vi "LoadCfgXMLFile.vi"(7 "ChassisType":T1, 8 "error in":errorcluster, 11 "XML File Path":path) -> (0 "error out":errorcluster, 3 "Chassis Cfg":refnum<class "ChassisCfg.lvclass">)   [LabVIEW 2012, in "Configuration Grandmaster.lvlib" / "ChassisCfg.lvclass"]
uses:
  ChassisCfg.lvclass
  Common/Controls/Chassis Type.ctl
  Common/Controls/LS Lock Sizes.ctl
  Custom Ctrls/Master CfgXML/ge_XMLHdr_TimingGrp.ctl
  Custom Ctrls/Master CfgXML/ge_XMLHdr_ChanGroups.ctl
  Custom Ctrls/Master Cfg/ge_GrpHdr.ctl
  Custom Ctrls/ge_MeasType.ctl
  ChassisCfg.lvclass/ChassisCfg.ctl
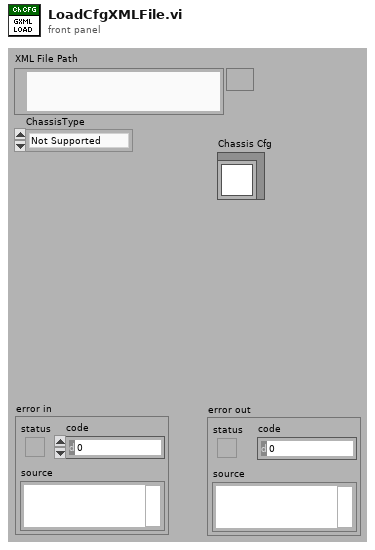
[diagram p1: front panel]
types:
  T1 = typedef "Chassis Type.ctl" = enum16{"Not Supported", "C Series 1-Slot", "C Series 4-Slot", "C Series 8-Slot", "PXI 8-Slot", "PXIe 18-Slot"}
  T2 = typedef "ge_XMLHdr_TimingGrp.ctl" = cluster{"Rate":dbl, "ReadBlk":i32, "Modbus URL":string, "ChanGroups":T3}
  T3 = typedef "ge_XMLHdr_ChanGroups.ctl" = T4[]
  T4 = typedef "ge_GrpHdr.ctl" = cluster{"GroupName":string, "MeasType":T5}
  T5 = typedef "ge_MeasType.ctl" = enum16{"Voltage", "Frequency", "Tachometer", "Dynamic", "Thermocouple", "RTD", "Strain", "Current", "Resistance"}
  T6 = typedef "LS Lock Sizes.ctl" = enum16{"No", "250ms", "500ms", "1s"}
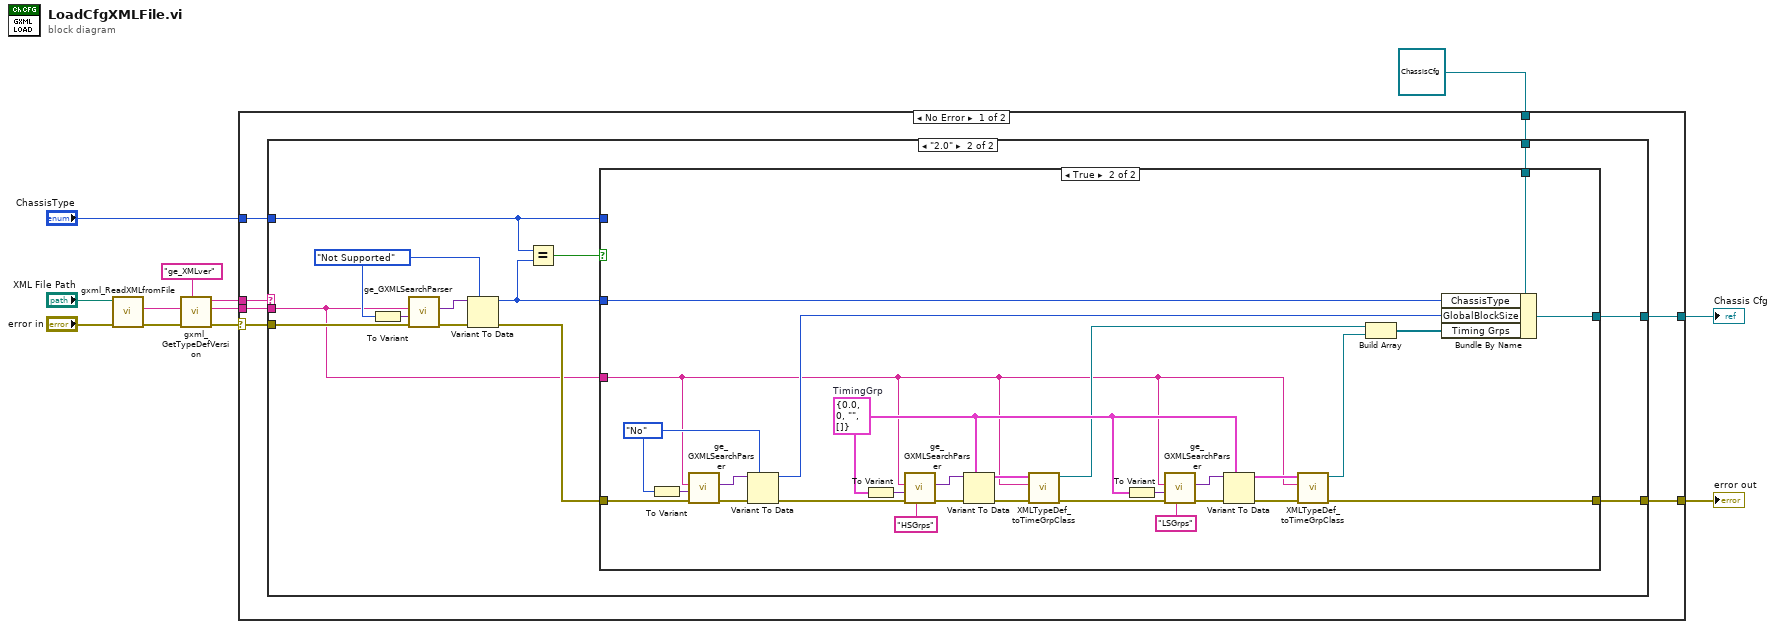
[diagram p0: block diagram]
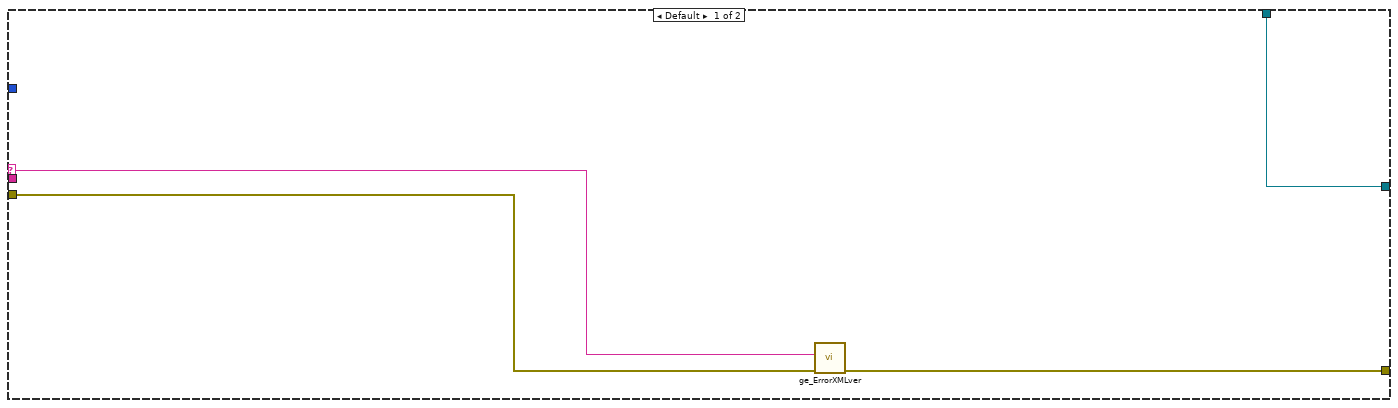
[diagram p2: hidden frame]
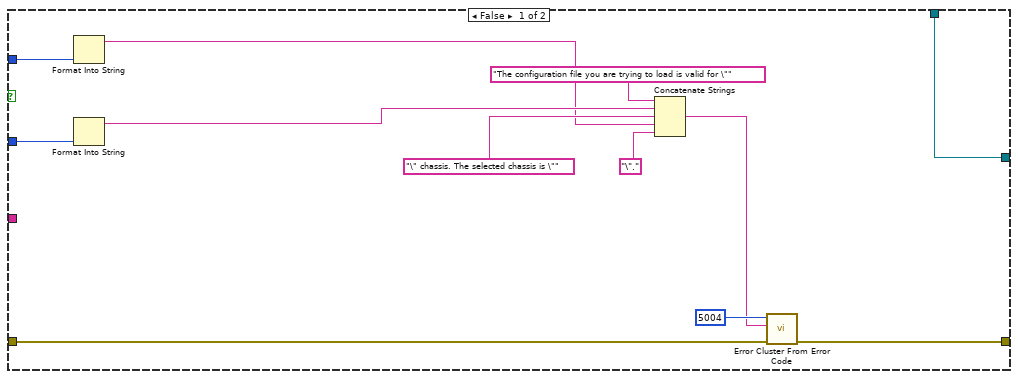
[diagram p3: hidden frame]
diagram:
  n1 = call <userlib>:"gxml_ReadXMLfromFile.vi"("error in"="error in", "XML File Path"="XML File Path") -> ("error out"=w8:errorcluster, "XML String Out"=w9:string)  [unwired: 7 in, 1 out]
  n2 = call <userlib>:"gxml_GetTypeDefVersion.vi"("Version Tag Name"="ge_XMLver", "error in"=w8, "XML String In"=w9) -> ("error out"=w5:errorcluster, "XML String Out"=w6:string, "Version String"=w4:string)  [unwired: 6 in]
  n3 = case shown="No Error" w5 {
    selector: w5 -> [w17 w79]
    tunnel: [w19 w78] -> w1
    tunnel: [w18 w79] -> w12
    tunnel: w6 -> [w14 _]
    tunnel: refnum<class "ChassisCfg.lvclass"> refnum ("Chassis Config") -> [w16 w78]
    tunnel: w4 -> [w15 _]
    tunnel: "ChassisType" -> [w13 _]
    frame No Error {
      n4 = case shown="\"2.0\"" w15 {
        selector: w15 -> [w20 _]
        tunnel: [w23 w36] -> w19
        tunnel: [w22 w35] -> w18
        tunnel: w17 -> [w21 w31]
        tunnel: w16 -> [w23 w34]
        tunnel: w14 -> [_ w27]
        tunnel: w13 -> [_ w25]
        frame Default {
          n5 = call "ge_ErrorXMLver.vi"("error in"=w21, "File Version Number"=w20) -> ("error out"=w22:errorcluster)  [unwired: 9 in]
        }
        frame "2.0" {
          w28 = Chassis_Type."Not Supported" ("ChassisType")
          n6 = To Variant(anything=w28) -> (Variant=w29:variant)
          n7 = call "ge_GXMLSearchParser.vi"("error in"=w31, "TypeDesc"=w29, "XML String In"=w27) -> ("error out"=w33:errorcluster, "Parsed Data"=w30:variant)  [unwired: 7 in]
          n8 = Variant To Data(error in=w33, type=w28, Variant=w30) -> (data=w24:T1, error out=w32:errorcluster)
          n9 = Equal?(x=w25, y=w24) -> (x = y?=w26:bool)
          n10 = case shown="True" w26 {
            tunnel: [w48 w77] -> w36
            tunnel: [w47 w50] -> w35
            tunnel: w34 -> [w48 w76]
            tunnel: w32 -> [w46 w75]
            tunnel: w24 -> [w43 w74]
            tunnel: w27 -> [_ w49]
            tunnel: w25 -> [w44 _]
            frame False {
              n11 = Format Into String(w44) -> (resulting string=w39:string)  [unwired: 3 in, 1 out]
              n12 = Format Into String(w43) -> (resulting string=w41:string)  [unwired: 3 in, 1 out]
              n13 = Concatenate Strings("The configuration file you are trying to load is valid for \"", w41, "\" chassis. The selected chassis is \"", w39, "\".") -> (w37:string)
              n14 = call <vilib>:"Error Cluster From Error Code.vi"("error in (no error)"=w46, "error message (\"\")"=w37, "error code (0)"=5004) -> ("error out"=w47:errorcluster)  [unwired: 6 in]
            }
            frame True {
              w59 = T2 {"Rate"=0.0, "ReadBlk"=0, "Modbus URL"="", "ChanGroups"=[]}  # TimingGrp
              w62 = LS_Lock_Sizes."No" ("GlobalBlockSize")
              n15 = To Variant(anything=w62) -> (Variant=w65:variant)
              n16 = call "ge_GXMLSearchParser.vi"("error in"=w75, "TypeDesc"=w65, "XML String In"=w49) -> ("error out"=w71:errorcluster, "Parsed Data"=w70:variant)  [unwired: 7 in]
              n17 = Variant To Data(error in=w71, type=w62, Variant=w70) -> (data=w61:T6, error out=w60:errorcluster)
              n18 = To Variant(anything=w59) -> (Variant=w63:variant)
              n19 = call "ge_GXMLSearchParser.vi"("String ID"="HSGrps", "error in"=w60, "TypeDesc"=w63, "XML String In"=w49) -> ("error out"=w69:errorcluster, "Parsed Data"=w68:variant)  [unwired: 6 in]
              n20 = Variant To Data(error in=w69, type=w59, Variant=w68) -> (data=w55:T2, error out=w56:errorcluster)
              n21 = call "XMLTypeDef_toTimeGrpClass.vi"("error in (no error)"=w56, "XML String"=w49, "TimingGrp"=w55) -> ("error out"=w54:errorcluster, "TimingGrp out"=w58:refnum<class "TimingGrp.lvclass">)  [unwired: 7 in]
              n22 = To Variant(anything=w59) -> (Variant=w64:variant)
              n23 = call "ge_GXMLSearchParser.vi"("String ID"="LSGrps", "error in"=w54, "TypeDesc"=w64, "XML String In"=w49) -> ("error out"=w66:errorcluster, "Parsed Data"=w67:variant)  [unwired: 6 in]
              n24 = Variant To Data(error in=w66, type=w59, Variant=w67) -> (data=w52:T2, error out=w53:errorcluster)
              n25 = call "XMLTypeDef_toTimeGrpClass.vi"("error in (no error)"=w53, "XML String"=w49, "TimingGrp"=w52) -> ("error out"=w50:errorcluster, "TimingGrp out"=w51:refnum<class "TimingGrp.lvclass">)  [unwired: 7 in]
              n26 = Build Array(w58, w51) -> (w57:refnum<class "TimingGrp.lvclass">[])
              n27 = Bundle By Name(cluster=w76, "ChassisType"=w74, "GlobalBlockSize"=w61, "Timing Grps"=w57) -> (w77:refnum<class "ChassisCfg.lvclass">)
            }
          }
        }
      }
    }
    frame Error {
    }
  }
  "Chassis Cfg" <- w1
  "error out" <- w12
